vi "MCP3008-TMP36.vi"() -> ()   [LabVIEW 2014]
uses:
  <vilib>/MakerHub/LINX/LMH-LINX.lvlib
  <vilib>/MakerHub/LINX/Public/Utilities/Open Local.vi
  <vilib>/MakerHub/LINX/Private/Type Defs/Peripherals/SPI/SPI CS Logic Level.ctl
  <vilib>/MakerHub/LINX/Public/Peripherals/SPI/SPI CS Config.ctl
  <vilib>/MakerHub/LINX/Private/Type Defs/Peripherals/SPI/SPI Bit Order.ctl
  <vilib>/MakerHub/LINX/Private/Type Defs/Peripherals/SPI/SPI Mode.ctl
  <vilib>/MakerHub/LINX/Private/Type Defs/Peripherals/SPI/SPI Configuration.ctl
panel:
  out "Temperature (degC)":dbl
  out "Converted Voltage (V)":dbl
  in  "Channel Select (CH0)":T1(ring)
  in  "Single-Diff Select (Diff)":enum16{"Differential", "Single-Ended"}(ring)
  out "10-bit ADC Code":u16 format="%.0x"
  in  "SPI Configuration":T2={"Clock Frequency"=1000000, "Bit Order"=enum."MSb First", "SPI Mode"=enum."Mode 0"}
  in  "CS Configuration":T5={"CS Channel"=7, "CS Logic Level"=enum."Active Low"}
  in  "stop":bool
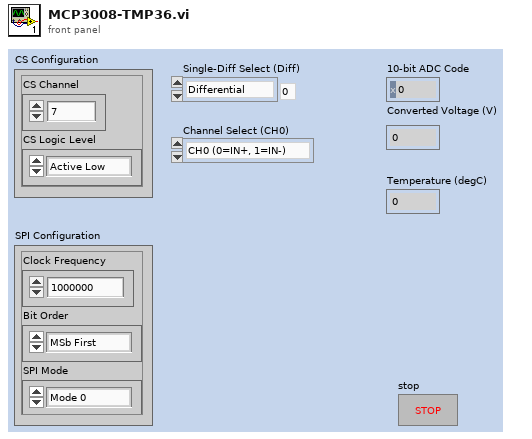
[diagram p1: front panel]
types:
  T1 = enum16{"CH0 (0=IN+, 1=IN-)", "CH1 (1=IN+, 0=IN-)", "CH2 (2=IN+, 3=IN-)", "CH3 (3=IN+, 2=IN-)", "CH4 (4=IN+, 5=IN-)", "CH5 (5=IN+, 4=IN-)", "CH6 (6=IN+, 7=IN-)", "CH7 (7=IN+, 6=IN-)"}
  T2 = typedef "LMH-LINX.lvlib/SPI Configuration.ctl" = cluster{"Clock Frequency":u32, "Bit Order":T3, "SPI Mode":T4}
  T3 = typedef "LMH-LINX.lvlib/SPI Bit Order.ctl" = enum8{"LSb First", "MSb First"}
  T4 = typedef "LMH-LINX.lvlib/SPI Mode.ctl" = enum8{"Mode 0", "Mode 1", "Mode 2", "Mode 3"}
  T5 = typedef "LMH-LINX.lvlib/SPI CS Config.ctl" = cluster{"CS Channel":u8, "CS Logic Level":T6}
  T6 = typedef "LMH-LINX.lvlib/SPI CS Logic Level.ctl" = enum8{"Active Low", "Active High"}
  T7 = typedef "LMH-LINX.lvlib/LINX Ref.ctl" = cluster{"IO":T8, "Interface":T9, "LINX Device Config":T10}
  T8 = typedef "LMH-LINX.lvlib/Platform.ctl" = enum16{"Remote", "Local"}
  T9 = typedef "LMH-LINX.lvlib/Interface.ctl" = enum16{"Serial", "TCP"}
  T10 = typedef "LMH-LINX.lvlib/Device.lvlib/LINX Device Config.ctl" = cluster{"Interface":T9, "COM Port":refnum<visa-resource-name>, "TCP Configuration":T11, "Device Family":u8, "Device ID":u8, "Device Name":string, "TCP Ref":refnum<k5>, "Channels":T12}
  T11 = typedef "LMH-LINX.lvlib/Device.lvlib/TCP Config.ctl" = cluster{"IP Address":string, "Port":u16}
  T12 = typedef "LMH-LINX.lvlib/Channels.ctl" = cluster{"DI":u8[], "DO":u8[], "AI":u8[], "AO":u8[], "PWM":u8[], "QE":u8[], "UART":u8[], "I2C 2":u8[], "SPI":u8[], "CAN":u8[], "Servo":u8[], "AI Ref (V)":dbl, "AI Resolution (Bits)":u8, "AO Ref (V)":dbl, "AO Resolution (Bits)":u8}
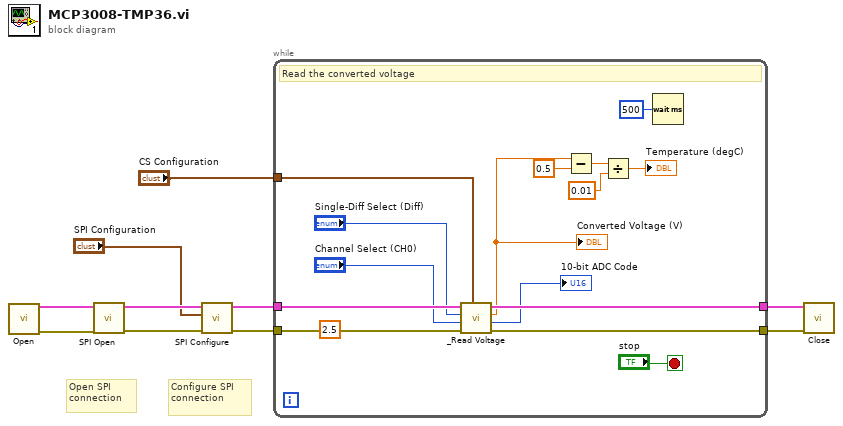
[diagram p0: block diagram]
diagram:
  # "Configure SPI connection"
  # "Open SPI connection"
  n1 = call-poly <vilib>:"Open.vi"() -> ("Error Out"=w3:errorcluster, "LINX Resource"=w4:T7)  [unwired: 9 in, 1 out]
  n2 = call <vilib>:"SPI Open.vi"("Error In"=w3, "LINX Resource"=w4) -> ("Error Out"=w5:errorcluster, "LINX Resource"=w6:T7)  [unwired: 8 in]
  n3 = call <vilib>:"SPI Configure.vi"("Error In"=w5, "SPI Configuration"="SPI Configuration", "LINX Resource"=w6) -> ("Error Out"=w7:errorcluster, "LINX Resource"=w8:T7)  [unwired: 6 in, 1 out]
  n4 = while {
    tunnel: w7 -> [w26]
    tunnel: w8 -> [w23]
    tunnel: [w24] -> w9
    tunnel: [w22] -> w10
    tunnel: "CS Configuration" -> [w21]
    stop <- "stop" stop-if-true
    # "Read the converted voltage"
    n5 = call "_Read Voltage.vi"("Vref (3.3V)"=2.5, "CS Configuration"=w21, "error in (no error)"=w26, "Channel Select (CH0)"="Channel Select (CH0)", "Single-Diff Select (Diff)"="Single-Diff Select (Diff)", "LINX Resource in"=w23) -> ("error out"=w24:errorcluster, "12-bit ADC Code"=→"10-bit ADC Code":u16, "Converted Voltage (V)"=w15:dbl, "LINX Resource out"=w22:T7)  [unwired: 2 in]
    "Converted Voltage (V)" <- w15
    n6 = Subtract(x=w15, y=0.5) -> (x-y=w13:dbl)
    n7 = Divide(x=w13, y=0.01) -> (x/y=→"Temperature (degC)":dbl)
    n8 = Wait (ms)(milliseconds to wait=u32 500) -> ()  [unwired: 1 out]
  }
  n9 = call <vilib>:"Close.vi"("Error In"=w9, "LINX Resource"=w10) -> ()  [unwired: 9 in, 1 out]
